vi "Connection.vi"(7 "ReadMode (Standard)":T1(ring), 8 "error in (no error)":errorcluster, 9 "Port":u16, 10 "Address":string, 11 "Connection":refnum<k5>) -> (0 "error out":errorcluster, 3 "Connection":refnum<class "Connection.lvclass">)   [LabVIEW 2021, in "TcpServer.lvlib" / "Connection.lvclass"]
uses:
  Connection.lvclass
  Connection.lvclass/Connection.ctl
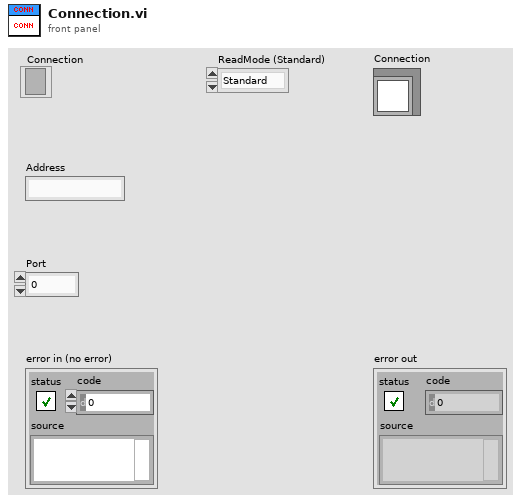
[diagram p1: front panel]
types:
  T1 = enum16{"Standard", "Buffered", "CRLF", "Immediate"}
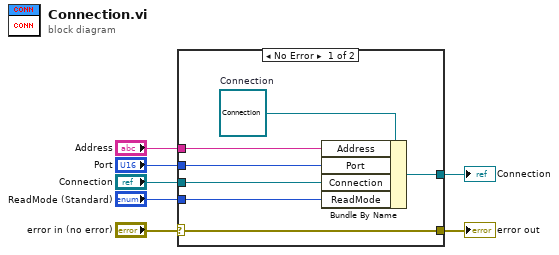
[diagram p0: block diagram]
diagram:
  n1 = case shown="No Error" "error in (no error)" {
    selector: "error in (no error)" -> [w14 w15]
    tunnel: [w14 w15] -> w6
    tunnel: [w13 _] -> w5
    tunnel: "Connection" -> [w12 _]
    tunnel: "Port" -> [w11 _]
    tunnel: "Address" -> [w10 _]
    tunnel: "ReadMode (Standard)" -> [w8 _]
    frame No Error {
      w9 = refnum<class "Connection.lvclass"> refnum  # Connection
      n2 = Bundle By Name(cluster=w9, "Address"=w10, "Port"=w11, "Connection"=w12, "ReadMode"=w8) -> (w13:refnum<class "Connection.lvclass">)
    }
    frame Error {
    }
  }
  "error out" <- w6
  "Connection" <- w5
